vi "Alarm_171213.vi"(0 "Enable":bool=TRUE, 5 "error in (no error)":errorcluster) -> (14 "CANCEL":bool caption="OK", 17 "minutes":dbl format="%#g", 18 "OK":bool, 19 "error out":errorcluster)   [LabVIEW 2016]
doc: "Displays a standard dialog box that prompts users to enter information, such as a user name and password.\n--------------------\n\nThis Express VI is configured as follows:\n\nMessage to Display to the User:Set an alarm signal if the mouse has not moved in the last\nThe inputs are: \nNumber: minutes"
panel:
  in  "Tab Control":enum32{"Page 1", "Page 2"}(tab)
  in  "OK1 2":bool caption="OK1"
  in  "OK1":bool
  out "String":string="Set an alarm signal if the mouse has not moved in the last"
  in  "minutes.":dbl caption="minutes" format="%#g"
  in  "Cancel":bool
  in  "OK2":bool
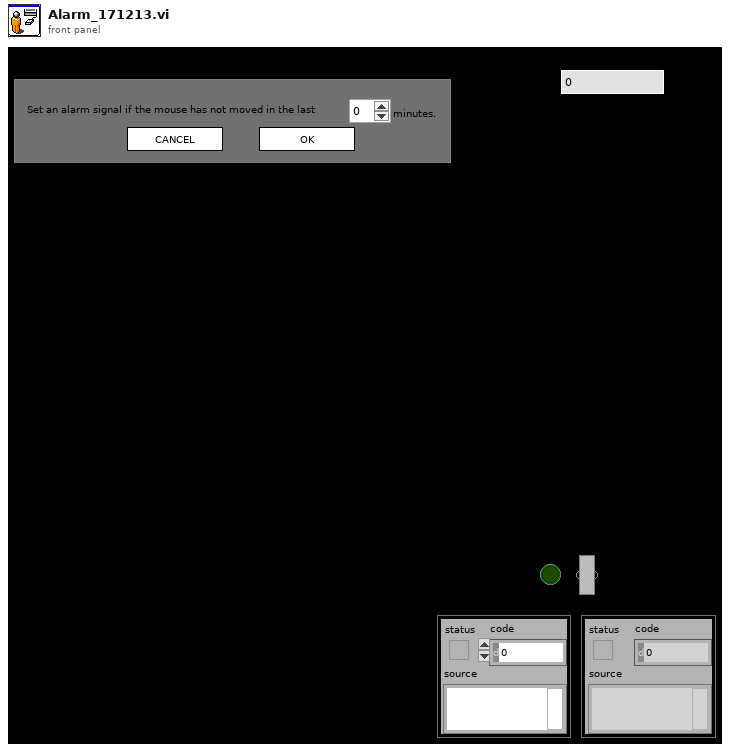
[diagram p1: front panel]
types:
  T1 = cluster{"Input Name":string, "Input Data Type":i32}[]
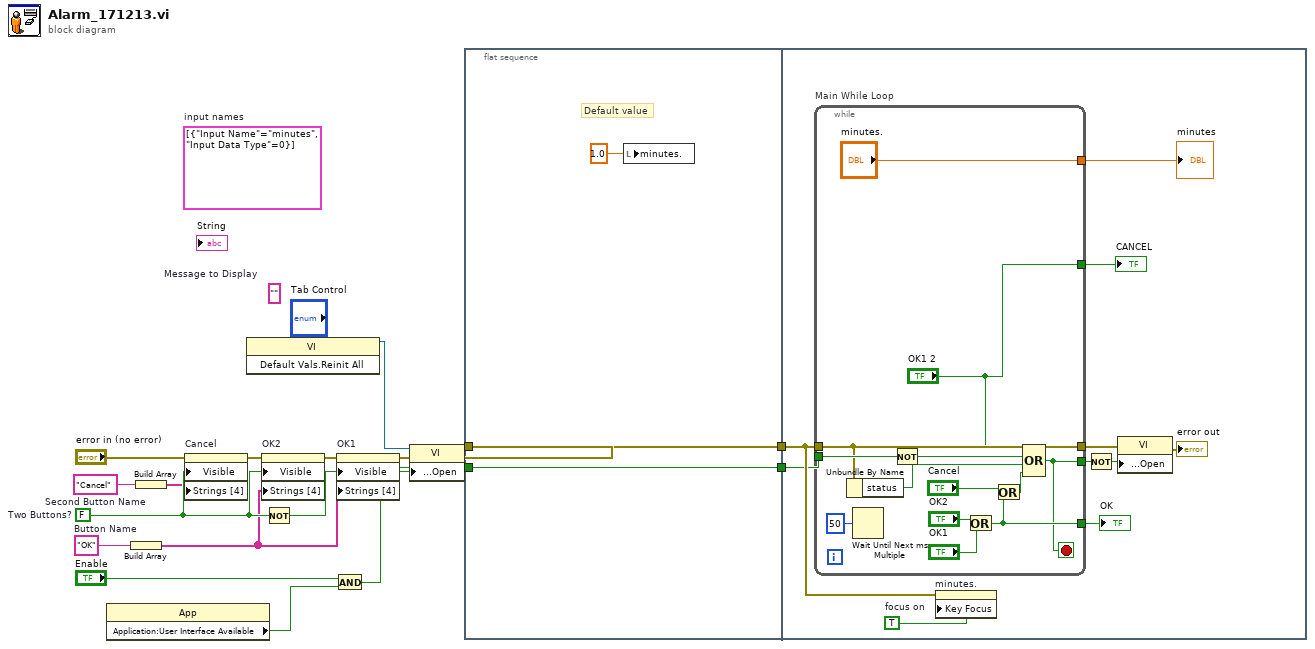
[diagram p0: block diagram]
diagram:
  (unwired) T1 [{"Input Name"="minutes", "Input Data Type"=0}]  # input names
  w12 = "Cancel"  # Second Button Name
  w10 = "OK"  # Button Name
  (unwired) ""  # Message to Display
  w17 = FALSE  # Two Buttons?
  n1 = property class="App"() -> ("Application:User Interface Available"=w4:bool)  [unwired: 2 in, 2 out]
  n2 = Build Array(w10) -> (w11:string[])
  n3 = Build Array(w12) -> (w13:string[])
  n4 = property on="Cancel" class="Bool"(error in="error in (no error)", "Visible"=w17, "Strings [4]"=w13) -> (error out=w15:errorcluster)  [unwired: 1 in, 1 out]
  n5 = invoke class="VI" method="Default Vals.Reinit All"() -> (reference out=w3:refnum<vi>)  [unwired: 3 in, 2 out]
  n6 = property on="OK2" class="Bool"(error in=w15, "Visible"=w17, "Strings [4]"=w11) -> (error out=w14:errorcluster)  [unwired: 1 in, 1 out]
  n7 = Not(x=w17) -> (.not. x?=w16:bool)
  n8 = And(x="Enable", y=w4) -> (x .and. y?=w5:bool)
  n9 = property on="OK1" class="Bool"(error in=w14, "Visible"=w16, "Strings [4]"=w11) -> (error out=w9:errorcluster)  [unwired: 1 in, 1 out]
  n10 = property class="VI"(reference=w3, error in=w9, "Front Panel Window:Open"=w5) -> (error out=w8:errorcluster)  [unwired: 1 out]
  n11 = flat-sequence {
    tunnel: w5 -> [w19]
    tunnel: w8 -> [w20]
    tunnel: [w20] -> w2
    tunnel: [w19] -> w1
    tunnel: w2 -> [w27]
    tunnel: w1 -> [w24]
    frame #0 {
      # "Default value"
      n12 = local write "minutes."(1.0 ("minutes.")) -> ()
    }
    frame #1 {
      w22 = TRUE  # focus on
      n13 = while "Main While Loop" {
        tunnel: [w40] -> w30
        tunnel: w24 -> [w38]
        tunnel: [w36] -> w28
        tunnel: w27 -> [w35]
        tunnel: [w35] -> w26
        tunnel: ["minutes."] -> w23
        tunnel: ["OK1 2"] -> w21
        stop <- w36 stop-if-true
        n14 = Unbundle By Name(w35) -> ("status"=w33:bool)
        n15 = Wait Until Next ms Multiple(millisecond multiple=u32 50) -> ()  [unwired: 1 out]
        n16 = Not(x=w38) -> (.not. x?=w37:bool)
        n17 = Or(x="OK2", y="OK1") -> (x .or. y?=w40:bool)
        n18 = Or(x="Cancel", y=w40) -> (x .or. y?=w34:bool)
        n19 = Compound Arithmetic op=OR("OK1 2", w37, w33, w34) -> (w36:bool)
      }
      "OK" <- w30
      "minutes" <- w23
      "CANCEL" <- w21
      n20 = property on="minutes." class="DigNum (strict)"(error in=w27, "Key Focus"=w22) -> ()  [unwired: 1 in, 2 out]
      n21 = Not(x=w28) -> (.not. x?=w29:bool)
      n22 = property class="VI"(error in=w26, "Front Panel Window:Open"=w29) -> (error out=→"error out":errorcluster)  [unwired: 1 in, 1 out]
    }
  }
